vi "1D Array of VArrays to MultiD Array.vi"(8 "error in (no error)":errorcluster, 9 "Element Type":variant, 10 "Array of VArrays":variant[](array[variant])) -> (0 "error out":errorcluster, 2 "MultiD Array":variant)   [LabVIEW 2020, in "openg_variant.lvlib"]
uses:
  openg_variant.lvlib
panel:
  # "EXPERIMENTAL"
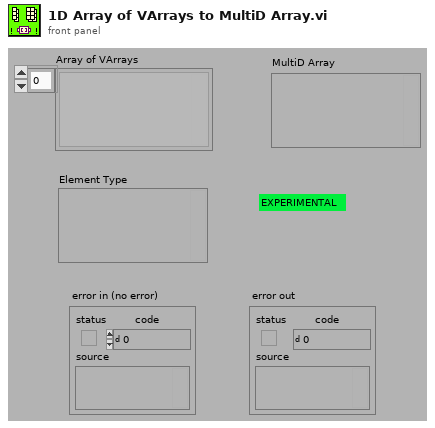
[diagram p1: front panel]
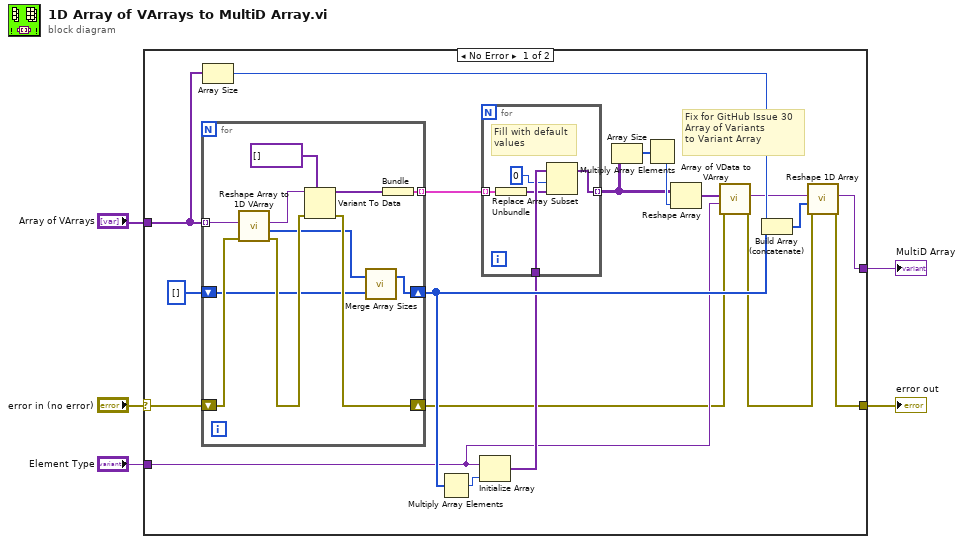
[diagram p0: block diagram]
diagram:
  n1 = case shown="No Error" "error in (no error)" {
    selector: "error in (no error)" -> [w24 w41]
    tunnel: [w20 w41] -> w5
    tunnel: [w17 _] -> w2
    tunnel: "Array of VArrays" -> [w23 _]
    tunnel: "Element Type" -> [w8 _]
    frame No Error {
      # "Fix for GitHub Issue 30\nArray of Variants\nto Variant Array"
      n2 = for {
        tunnel: w23 -> [w40] mode=indexing
        shift-right: [w36] -> w7
        shift-left: w24 -> [w39]
        tunnel: [w30] -> w15 mode=indexing
        shift-right: [w32] -> w13
        shift-left: i32[] [] -> [w33]
        n3 = call "Reshape Array to 1D VArray.vi"("error in (no error)"=w39, "MultiD Array"=w40) -> ("error out"=w37:errorcluster, "Size(s)"=w31:u32[], "1D VArray"=w38:variant)  [unwired: 7 in]
        n4 = Variant To Data(error in=w37, type=variant[] [], Variant=w38) -> (data=w34:variant[], error out=w36:errorcluster)
        n5 = call "Merge Array Sizes.vi"("Sizes 2"=w33, "Sizes"=w31) -> ("Sizes out"=w32:i32[])  [unwired: 1 in]
        n6 = Bundle(w34) -> (w30:cluster{variant[]})  [unwired: 1 in]
      }
      n7 = Array Size(array=w23) -> (size(s)=w19:i32)
      n8 = Multiply Array Elements(1:w13) -> (0:w12:i32)
      n9 = Initialize Array(w8, w12) -> (w11:variant[])
      n10 = for {
        tunnel: w15 -> [w29] mode=indexing
        tunnel: [w28] -> w14 mode=indexing
        tunnel: w11 -> [w27]
        # "Fill with default\nvalues"
        n11 = Unbundle(w29) -> (w26:variant[])
        n12 = Replace Array Subset(array=w27, new element=w26, index=0) -> (w28:variant[])
      }
      n13 = Array Size(array=w14) -> (size(s)=w22:i32[])
      n14 = Multiply Array Elements(1:w22) -> (0:w21:i32)
      n15 = Reshape Array(w14, w21) -> (w10:variant[])
      n16 = call "Array of VData to VArray.vi"("error in (no error)"=w7, "Element Type (when empty)"=w8, "1D Array of VData"=w10) -> ("error out"=w6:errorcluster, "VArray"=w9:variant)  [unwired: 7 in]
      n17 = Build Array (concatenate)(w19, w13) -> (w18:i32[])
      n18 = call "Reshape 1D Array.vi"("error in (no error)"=w6, "Size(s)"=w18, "1D Array"=w9) -> ("error out"=w20:errorcluster, "Reshaped VArray"=w17:variant)  [unwired: 7 in]
    }
    frame Error {
    }
  }
  "error out" <- w5
  "MultiD Array" <- w2
